vi "Open Video Writer.vi"(0 "video writer in":refnum<class "MSC Video Writer.lvclass">, 5 "error in (no error)":errorcluster) -> (14 "video writer out":refnum<class "MSC Video Writer.lvclass">, 19 "error out":errorcluster)   [LabVIEW 2014, in "MSC Video Writer.lvclass"]
uses:
  MSC Video Writer.lvclass
  MSC Video Writer.lvclass/MSC Video Writer.ctl
  MSC Image_class/controls/Image Type.ctl
  Dependencies/x86/MSC I Process32.dll
  MSC Image_class/MSC Image.lvclass
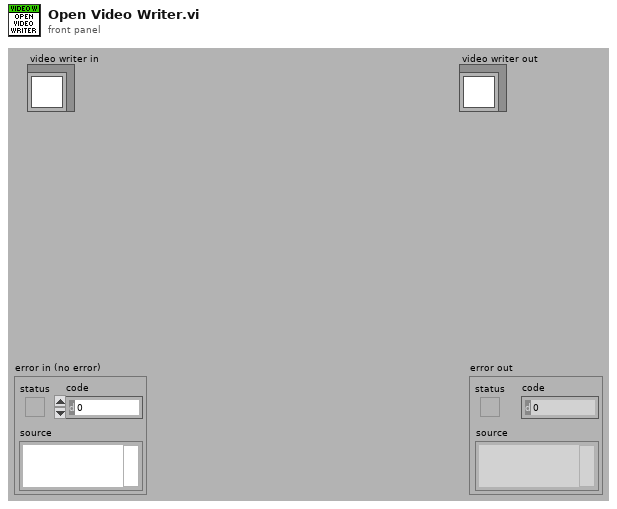
[diagram p1: front panel]
types:
  T1 = typedef "MSC Video Writer.lvclass/Video Writer.ctl" = cluster{"Pointer":u64, "FPS":u32, "Path":path, "FourCC Codec":string, "Size":T2, "Type":T3}
  T2 = typedef "MSC Image.lvclass/Size.ctl" = cluster{"Cols":i32, "Rows":i32}
  T3 = typedef "MSC Image.lvclass/Image Type.ctl" = i32
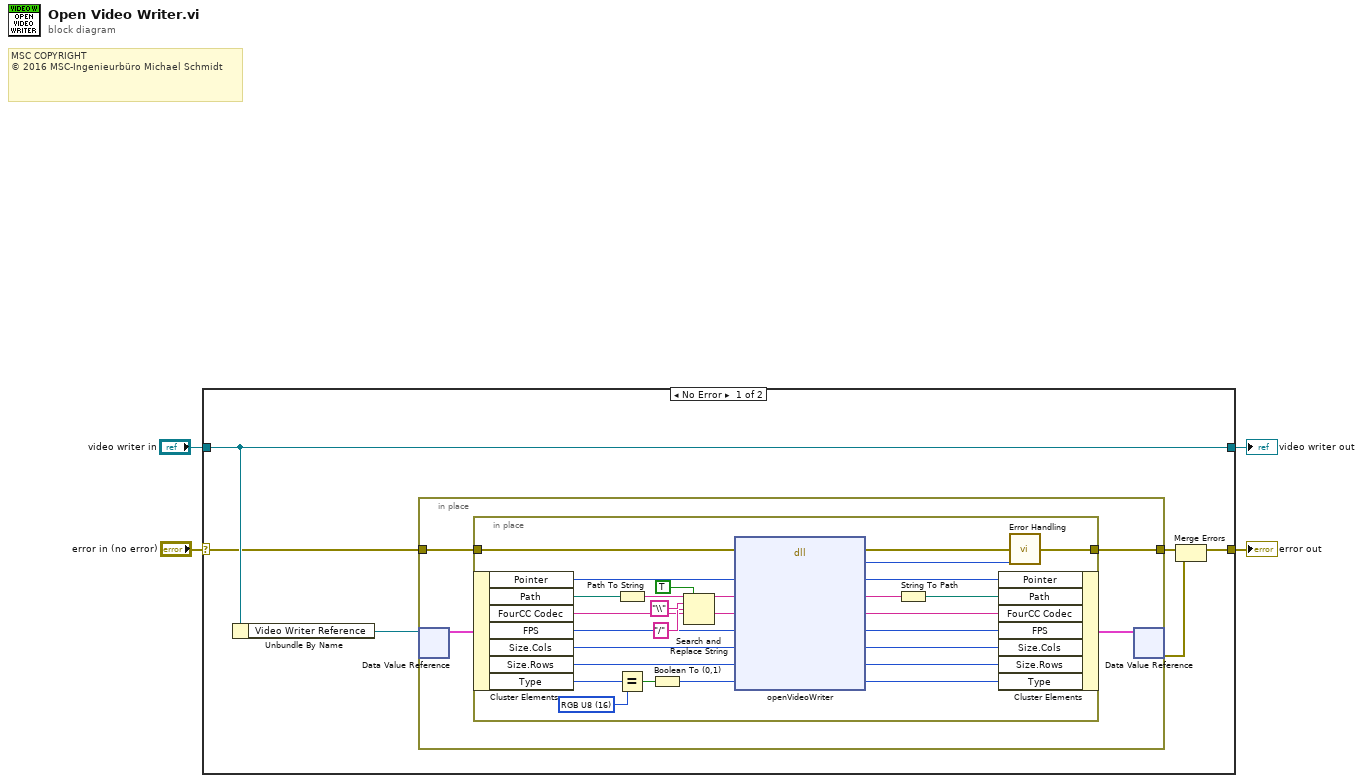
[diagram p0: block diagram]
diagram:
  # "MSC COPYRIGHT\n© 2016 MSC-Ingenieurbüro Michael Schmidt"
  # "MSC COPYRIGHT\n© 2016 MSC-Ingenieurbüro Michael Schmidt"
  n1 = case shown="No Error" "error in (no error)" {
    selector: "error in (no error)" -> [w6 w42]
    tunnel: [w5 w42] -> w3
    tunnel: [w10 w41] -> w1
    tunnel: "video writer in" -> [w10 w41]
    frame No Error {
      n2 = Unbundle By Name(w10) -> ("Video Writer Reference"=w7:refnum<data-value>)
      n3 = in-place {
        in-place-border: [w12] -> w8
        in-place-border: w6 -> [w11]
        n4 = in-place-dvr #1(w7) -> (w13:T1)  [unwired: 1 out]
        n5 = in-place {
          in-place-border: [w37] -> w12
          in-place-border: w11 -> [w40]
          w18 = T3 16 items=["Grayscale U8"=0, "Grayscale U16"=2, "Grayscale Single"=5, "Grayscale Double"=6, "RGB U8"=16] ("y")
          n6 = in-place-cluster #2(w13) -> ("Pointer"=w36:u64, "Path"=w30:path, "FourCC Codec"=w28:string, "FPS"=w27:u32, "Size.Cols"=w24:i32, "Size.Rows"=w23:i32, "Type"=w15:T3)
          n7 = Path To String(path=w30) -> (string=w31:string)
          n8 = Equal?(x=w15, y=w18) -> (x = y?=w17:bool)
          n9 = Boolean To (0,1)(Boolean=w17) -> (0, 1=w16:i16)
          n10 = Search and Replace String(replace all?=TRUE ("replace all? (F)"), input string=w31, search string="\\", replace string="/" ("replace string (\"\")")) -> (result string=w29:string)  [unwired: 4 in, 3 out]
          n11 = dll-call lib="C:/Users/MSC/LabVIEW Projekte/LV 2014/MSC I-Process/user.lib/MSC-I Process/Dependencies/x86/MSC I Process*.dll" fn="openVideoWriter"(error in=w40, "writerPointer"=w36, "pathString"=w29, "fourccString"=w28, "fps"=w27, "cols"=w24, "rows"=w23, "colorType"=w16) -> (error out=w38:errorcluster, "error"=w39:i32, "writerPointer"=w35:u64, "pathString"=w20:string, "fourccString"=w22:string, "fps"=w19:u32, "cols"=w26:i32, "rows"=w25:i32)  [unwired: 3 in, 1 out]
          n12 = String To Path(string=w20) -> (path=w21:path)
          n13 = in-place-cluster #2("Pointer"=w35, "Path"=w21, "FourCC Codec"=w22, "FPS"=w19, "Size.Cols"=w26, "Size.Rows"=w25, "Type"=w15) -> (w14:T1)
          n14 = call "Error Handling.vi"("error in (no error)"=w38, "return type"=w39) -> ("error out"=w37:errorcluster)  [unwired: 12 in, 1 out]
        }
        n15 = in-place-dvr #1(w14) -> (w9:errorcluster)  [unwired: 1 out]
      }
      n16 = Merge Errors(w8, w9) -> (w5:errorcluster)
    }
    frame Error {
    }
  }
  "error out" <- w3
  "video writer out" <- w1
